vi "rsidr_core_global.vi"() -> ()   [LabVIEW 2020, in "Rohde&Schwarz RTx Oscilloscopes.lvlib"] (continued)
reference waveforms of all active channels, and activates the references. This action works only with single acquisition.\nThe channels are assigned to the references: C1 to R1, C2 to R2 and so on. If a channel is off, the assigned reference is also not active.\n\nAvailable Repeated Capabilities:\nNone\n\nRemote-control command(s):\nTRIGger:EVENt:REFSave"}, {"Level"=3, "Class Only"=FALSE, "Identifier"="RSRTX_ATTR_ACTIONS_ON_TRIGGER_PULSE_OUT", "Descriptive Name"="Actions On Trigger Pulse Out", "Data Type"=3, "Command"="TRIG:EVEN:TRIG", "Access"=2, "Range Table"="", "Read Callback"="", "Write Callback"="", "Supported Models"="", "Instrument Options"="", "Flags"=0, "Help"="If ON, the instrument generates a pulse on the Aux Out connector on trigger event. The acquisition is not delayed, the pulse generation runs asynchronously.\nTo set the pulse width and polarity of the trigger out pulse, use:\nRSRTX_ATTR_TRIGGER_OUT_PULSE_WIDTH\nRSRTX_ATTR_TRIGGER_OUT_POLARITY\n\nAvailable Repeated Capabilities:\nNone\n\nRemote-control command(s):\nTRIGger:EVENt:TRIGgerout"}, {"Level"=2, "Class Only"=TRUE, "Identifier"="", "Descriptive Name"="Trigger Out", "Data Type"=0, "Command"="", "Access"=0, "Range Table"="", "Read Callback"="", "Write Callback"="", "Supported Models"="", "Instrument Options"="", "Flags"=0, "Help"="Atributes configures the Trigger Out."}, {"Level"=3, "Class Only"=FALSE, "Identifier"="RSRTX_ATTR_TRIGGER_OUT_MODE", "Descriptive Name"="Trigger Out Mode", "Data Type"=0, "Command"="TRIG:OUT:MODE", "Access"=2, "Range Table"="rsrtx_rngTriggerOutMode", "Read Callback"="", "Write Callback"="", "Supported Models"="", "Instrument Options"="", "Flags"=0, "Help"="Defines wether and when a trigger out pulse is generated: never, on trigger event, or on mask violation.\n\nAvailable Repeated Capabilities:\nNone\n\nRemote-control command(s):\nTRIGger:OUT:MODE"}, {"Level"=3, "Class Only"=FALSE, "Identifier"="RSRTX_ATTR_TRIGGER_OUT_POLARITY", "Descriptive Name"="Trigger Out Polarity", "Data Type"=0, "Command"="TRIG:OUT:POL", "Access"=2, "Range Table"="rsrtx_rngPolarity", "Read Callback"="", "Write Callback"="", "Supported Models"="", "Instrument Options"="", "Flags"=0, "Help"="Sets the polarity of the trigger out pulse.\n\nAvailable Repeated Capabilities:\nNone\n\nRemote-control command(s):\nTRIGger:OUT:POLarity"}, {"Level"=3, "Class Only"=FALSE, "Identifier"="RSRTX_ATTR_TRIGGER_OUT_PULSE_WIDTH", "Descriptive Name"="Trigger Out Pulse Width", "Data Type"=1, "Command"="TRIG:OUT:PLEN", "Access"=2, "Range Table"="", "Read Callback"="", "Write Callback"="", "Supported Models"="", "Instrument Options"="", "Flags"=0, "Help"="Defines the pulse width of the trigger out pulse.\n\nAvailable Repeated Capabilities:\nNone\n\nRemote-control command(s):\nTRIGger:OUT:PLENgth"}, {"Level"=2, "Class Only"=TRUE, "Identifier"="", "Descriptive Name"="Runt", "Data Type"=0, "Command"="", "Access"=0, "Range Table"="", "Read Callback"="", "Write Callback"="", "Supported Models"="", "Instrument Options"="", "Flags"=0, "Help"="A runt is a pulse lower than normal in amplitude. The amplitude crosses the first\nthreshold twice in succession without crossing the second one. For example, this trig-\nger can detect logic, digital, and analog signals remaining below a specified threshold\namplitude because I/O ports are in undefined state."}, {"Level"=3, "Class Only"=FALSE, "Identifier"="RSRTX_ATTR_RUNT_TRIGGER_POLARITY", "Descriptive Name"="Runt Trigger Polarity", "Data Type"=0, "Command"="TRIG:A:RUNT:POL", "Access"=2, "Range Table"="rsrtx_rngPolarity", "Read Callback"="", "Write Callback"="", "Supported Models"="RTM|RTA", "Instrument Options"="", "Flags"=0, "Help"="Sets the polarity of a pulse, that is the direction of the first pulse slope.\n\nAvailable Repeated Capabilities:\nNone\n\nRemote-control command(s):\nTRIGger:A:RUNT:POLarity"}, {"Level"=3, "Class Only"=FALSE, "Identifier"="RSRTX_ATTR_RUNT_TRIGGER_WIDTH", "Descriptive Name"="Runt Trigger Width", "Data Type"=1, "Command"="TRIG:A:RUNT:WIDT", "Access"=2, "Range Table"="", "Read Callback"="", "Write Callback"="", "Supported Models"="RTM|RTA", "Instrument Options"="", "Flags"=0, "Help"="For the ranges WITHin and OUTSide, the <Time1> defines the center of a range which is defined by the limits +-<Delta>. For the ranges SHORter and LONGer, the width defines the maximum and minimum pulse width, respectively.\n\nAvailable Repeated Capabilities:\nNone\n\nRemote-control command(s):\nTRIGger:A:RUNT:WIDTh"}, {"Level"=3, "Class Only"=FALSE, "Identifier"="RSRTX_ATTR_RUNT_TRIGGER_DELTA", "Descriptive Name"="Runt Trigger Delta", "Data Type"=1, "Command"="TRIG:A:RUNT:DELT", "Access"=2, "Range Table"="", "Read Callback"="", "Write Callback"="", "Supported Models"="RTM|RTA", "Instrument Options"="", "Flags"=0, "Help"="Defines a range around the width value.\n\nAvailable Repeated Capabilities:\nNone\n\nRemote-control command(s):\nTRIGger:A:RUNT:DELTa"}, {"Level"=3, "Class Only"=FALSE, "Identifier"="RSRTX_ATTR_RUNT_TRIGGER_RANGE", "Descriptive Name"="Runt Trigger Range", "Data Type"=0, "Command"="TRIG:A:RUNT:RANG", "Access"=2, "Range Table"="rsrtx_rngWidthCondition", "Read Callback"="", "Write Callback"="", "Supported Models"="RTM|RTA", "Instrument Options"="", "Flags"=0, "Help"="Defines how the measured pulse width is compared with the given limit(s).\n\nAvailable Repeated Capabilities:\nNone\n\nRemote-control command(s):\nTRIGger:A:RUNT:RANGe"}, {"Level"=3, "Class Only"=TRUE, "Identifier"="", "Descriptive Name"="Channel", "Data Type"=0, "Command"="", "Access"=0, "Range Table"="", "Read Callback"="", "Write Callback"="", "Supported Models"="", "Instrument Options"="", "Flags"=0, "Help"="Attributes with channel repcap."}, {"Level"=4, "Class Only"=FALSE, "Identifier"="RSRTX_ATTR_RUNT_TRIGGER_LOWER_LEVEL", "Descriptive Name"="Runt Trigger Lower Level", "Data Type"=1, "Command"="TRIG:A:LEV{Channel}:RUNT:LOW", "Access"=2, "Range Table"="", "Read Callback"="", "Write Callback"="", "Supported Models"="RTM|RTA", "Instrument Options"="", "Flags"=0, "Help"="Set the lower voltage threshold. The instrument triggers if the amplitude crosses the first threshold twice in succession without crossing the second one.\n\nAvailable Repeated Capabilities:\nChannel: CH0, CH1, CH2, CH3, CH4, CHExt\r\n\nRemote-control command(s):\nTRIGger:A:LEVel<n>:RUNT:LOWer"}, {"Level"=4, "Class Only"=FALSE, "Identifier"="RSRTX_ATTR_RUNT_TRIGGER_UPPER_LEVEL", "Descriptive Name"="Runt Trigger Upper Level", "Data Type"=1, "Command"="TRIG:A:LEV{Channel}:RUNT:UPP", "Access"=2, "Range Table"="", "Read Callback"="", "Write Callback"="", "Supported Models"="RTM|RTA", "Instrument Options"="", "Flags"=0, "Help"="Set the upper voltage threshold. The instrument triggers if the amplitude crosses the first threshold twice in succession without crossing the second one.\n\nAvailable Repeated Capabilities:\nChannel: CH0, CH1, CH2, CH3, CH4, CHExt\r\n\nRemote-control command(s):\nTRIGger:A:LEVel<n>:RUNT:UPPer"}, {"Level"=2, "Class Only"=TRUE, "Identifier"="", "Descriptive Name"="Timeout", "Data Type"=0, "Command"="", "Access"=0, "Range Table"="", "Read Callback"="", "Write Callback"="", "Supported Models"="", "Instrument Options"="", "Flags"=0, "Help"="Configures the timeout trigger."}, {"Level"=3, "Class Only"=FALSE, "Identifier"="RSRTX_ATTR_TIMEOUT_TRIGGER_TIME", "Descriptive Name"="Timeout Trigger Time", "Data Type"=1, "Command"="TRIG:A:TIM:TIME", "Access"=2, "Range Table"="RsRtx_rngTimeoutTriggerTime", "Read Callback"="", "Write Callback"="", "Supported Models"="", "Instrument Options"="", "Flags"=0, "Help"="Sets the time limit for the timeout at which the instrument triggers.\n\nAvailable Repeated Capabilities:\nNone\n\nRemote-control command(s):\nTRIGger:A:TIMeout:TIME"}, {"Level"=3, "Class Only"=FALSE, "Identifier"="RSRTX_ATTR_TIMEOUT_TRIGGER_RANGE", "Descriptive Name"="Timeout Trigger Range", "Data Type"=0, "Command"="TRIG:A:TIM:RANG", "Access"=2, "Range Table"="RsRtx_rngTimeoutRange", "Read Callback"="", "Write Callback"="", "Supported Models"="", "Instrument Options"="", "Flags"=0, "Help"="Sets the relation of the signal level to the threshold.\n\nAvailable Repeated Capabilities:\nNone\n\nRemote-control command(s):\nTRIGger:A:TIMeout:RANGe"}, {"Level"=2, "Class Only"=TRUE, "Identifier"="", "Descriptive Name"="I2C", "Data Type"=0, "Command"="", "Access"=0, "Range Table"="", "Read Callback"="", "Write Callback"="", "Supported Models"="", "Instrument Options"="", "Flags"=0, "Help"="Atributes configures the Trigger for I2C protocol."}, {"Level"=3, "Class Only"=FALSE, "Identifier"="RSRTX_ATTR_PROTOCOL_I2C_TRIGGER_ACCESS", "Descriptive Name"="Protocol I2C Trigger Access", "Data Type"=0, "Command"="TRIG:A:I2C:ACC", "Access"=2, "Range Table"="rsrtx_rngProtocolI2CAccessBit", "Read Callback"="", "Write Callback"="", "Supported Models"="", "Instrument Options"="", "Flags"=0, "Help"="Toggles the trigger condition between Read and Write access of the master.\n\nAvailable Repeated Capabilities:\nNone\n\nRemote-control command(s):\nTRIGger:A:I2C:ACCess"}, {"Level"=3, "Class Only"=FALSE, "Identifier"="RSRTX_ATTR_PROTOCOL_I2C_TRIGGER_ADDRESS_TYPE", "Descriptive Name"="Protocol I2C Trigger Address Type", "Data Type"=0, "Command"="TRIG:A:I2C:AMOD", "Access"=2, "Range Table"="rsrtx_rngAddressLength", "Read Callback"="", "Write Callback"="", "Supported Models"="", "Instrument Options"="", "Flags"=0, "Help"="Sets the lenght of the slave address.\n\nAvailable Repeated Capabilities:\nNone\n\nRemote-control command(s):\nTRIGger:A:I2C:AMODe"}, {"Level"=3, "Class Only"=FALSE, "Identifier"="RSRTX_ATTR_PROTOCOL_I2C_TRIGGER_ADDRESS", "Descriptive Name"="Protocol I2C Trigger Address", "Data Type"=2, "Command"="TRIG:A:I2C:ADDR", "Access"=2, "Range Table"="", "Read Callback"="", "Write Callback"="", "Supported Models"="", "Instrument Options"="", "Flags"=0, "Help"="Sets the address of the slave device. The address can have 7 bits or 10 bits.\n\nAvailable Repeated Capabilities:\nNone\n\nRemote-control command(s):\nTRIGger:A:I2C:ADDRess"}, {"Level"=3, "Class Only"=FALSE, "Identifier"="RSRTX_ATTR_PROTOCOL_I2C_TRIGGER_MODE", "Descriptive Name"="Protocol I2C Trigger Mode", "Data Type"=0, "Command"="TRIG:A:I2C:MODE", "Access"=2, "Range Table"="rsrtx_rngProtocolI2CTriggerType", "Read Callback"="", "Write Callback"="", "Supported Models"="", "Instrument Options"="", "Flags"=0, "Help"="Specifies the trigger mode for I2C.\n\nAvailable Repeated Capabilities:\nNone\n\nRemote-control command(s):\nTRIGger:A:I2C:MODE"}, {"Level"=3, "Class Only"=FALSE, "Identifier"="RSRTX_ATTR_PROTOCOL_I2C_TRIGGER_CONDITION_LENGTH", "Descriptive Name"="Protocol I2C Trigger Condition Length", "Data Type"=0, "Command"="TRIG:A:I2C:PLEN", "Access"=2, "Range Table"="rsrtx_rngProtocolI2CPatternLength", "Read Callback"="", "Write Callback"="", "Supported Models"="", "Instrument Options"="", "Flags"=0, "Help"="Defines how many bytes are considered in the trigger condition. To set the pattern for these bytes, use RSRTX_ATTR_PROTOCOL_I2C_TRIGGER_BIT_PATTERN.\n\nAvailable Repeated Capabilities:\nNone\n\nRemote-control command(s):\nTRIGger:A:I2C:PLENgth"}, {"Level"=3, "Class Only"=FALSE, "Identifier"="RSRTX_ATTR_PROTOCOL_I2C_TRIGGER_BIT_PATTERN", "Descriptive Name"="Protocol I2C Trigger Bit Pattern", "Data Type"=2, "Command"="TRIG:A:I2C:PATT", "Access"=2, "Range Table"="", "Read Callback"="", "Write Callback"="", "Supported Models"="", "Instrument Options"="", "Flags"=0, "Help"="Defines the bit pattern as trigger condition. Make sure that the correct pattern length has been defined before with RSRTX_ATTR_PROTOCOL_I2C_TRIGGER_CONDITION_LENGTH. SBinary pattern with max. 24 bit. Characters 0, 1, and X are allowed.\n\nAvailable Repeated Capabilities:\nNone\n\nRemote-control command(s):\nTRIGger:A:I2C:PATTern"}, {"Level"=3, "Class Only"=FALSE, "Identifier"="RSRTX_ATTR_PROTOCOL_I2C_TRIGGER_FIRST_BYTE_OFFSET", "Descriptive Name"="Protocol I2C Trigger First Byte Offset", "Data Type"=0, "Command"="TRIG:A:I2C:POFF", "Access"=2, "Range Table"="rsrtx_rngFirstBitOffset", "Read Callback"="", "Write Callback"="", "Supported Models"="", "Instrument Options"="", "Flags"=0, "Help"="Sets the number of bytes before the first byte of interest, relating to the end of the address bytes.\n\nAvailable Repeated Capabilities:\nNone\n\nRemote-control command(s):\nTRIGger:A:I2C:POFFset"}, {"Level"=2, "Class Only"=TRUE, "Identifier"="", "Descriptive Name"="SPI", "Data Type"=0, "Command"="", "Access"=0, "Range Table"="", "Read Callback"="", "Write Callback"="", "Supported Models"="", "Instrument Options"="", "Flags"=0, "Help"="Atributes configures the Trigger for SPI protocol."}, {"Level"=3, "Class Only"=FALSE, "Identifier"="RSRTX_ATTR_PROTOCOL_SPI_TRIGGER_MODE", "Descriptive Name"="Protocol SPI Trigger Mode", "Data Type"=0, "Command"="TRIG:A:SPI:MODE", "Access"=2, "Range Table"="rsrtx_rngProtocolSPITriggerType", "Read Callback"="", "Write Callback"="", "Supported Models"="", "Instrument Options"="", "Flags"=0, "Help"="Specifies the trigger mode for SPI/SSPI protocols.\n\nAvailable Repeated Capabilities:\nNone\n\nRemote-control command(s):\nTRIGger:A:SPI:MODE"}, {"Level"=3, "Class Only"=FALSE, "Identifier"="RSRTX_ATTR_PROTOCOL_SPI_TRIGGER_SOURCE", "Descriptive Name"="Protocol SPI Trigger Source", "Data Type"=0, "Command"="TRIG:A:SOUR:SPI", "Access"=2, "Range Table"="rsrtx_rngProtocolSPITriggerSource", "Read Callback"="", "Write Callback"="", "Supported Models"="RTM|RTA", "Instrument Options"="", "Flags"=0, "Help"="Selects the trigger source.\n\nAvailable Repeated Capabilities:\nNone\n\nRemote-control command(s):\nTRIGger:A:SOURce:SPI"}, {"Level"=3, "Class Only"=FALSE, "Identifier"="RSRTX_ATTR_PROTOCOL_SPI_TRIGGER_OFFSET", "Descriptive Name"="Protocol SPI Trigger Offset", "Data Type"=0, "Command"="TRIG:A:SPI:POFF", "Access"=2, "Range Table"="rsrtx_rngFirstBitOffset", "Read Callback"="", "Write Callback"="", "Supported Models"="", "Instrument Options"="", "Flags"=0, "Help"="Sets the number of bits before the first bit of the pattern.\n\nAvailable Repeated Capabilities:\nNone\n\nRemote-control command(s):\nTRIGger:A:SPI:POFFset"}, {"Level"=3, "Class Only"=FALSE, "Identifier"="RSRTX_ATTR_PROTOCOL_SPI_BIT_PATTERN_LENGTH", "Descriptive Name"="Protocol SPI Bit Pattern Length", "Data Type"=0, "Command"="TRIG:A:SPI:PLEN", "Access"=2, "Range Table"="rsrtx_rngSPIWordLength", "Read Callback"="", "Write Callback"="", "Supported Models"="", "Instrument Options"="", "Flags"=0, "Help"="Defines how many bits build up the serial pattern.\n\nAvailable Repeated Capabilities:\nNone\n\nRemote-control command(s):\nTRIGger:A:SPI:PLENgth"}, {"Level"=3, "Class Only"=FALSE, "Identifier"="RSRTX_ATTR_PROTOCOL_SPI_BIT_PATTERN", "Descriptive Name"="Protocol SPI Bit Pattern", "Data Type"=2, "Command"="TRIG:A:SPI:PATT", "Access"=2, "Range Table"="", "Read Callback"="", "Write Callback"="", "Supported Models"="", "Instrument Options"="", "Flags"=0, "Help"="Defines the bit pattern as trigger condition. The pattern length is adjusted to the number of bits defined in the pattern.\n\nAvailable Repeated Capabilities:\nNone\n\nRemote-control command(s):\nTRIGger:A:SPI:PATTern"}, {"Level"=2, "Class Only"=TRUE, "Identifier"="", "Descriptive Name"="UART", "Data Type"=0, "Command"="", "Access"=0, "Range Table"="", "Read Callback"="", "Write Callback"="", "Supported Models"="", "Instrument Options"="", "Flags"=0, "Help"="Atributes configures the Trigger for UART protocol."}, {"Level"=3, "Class Only"=FALSE, "Identifier"="RSRTX_ATTR_PROTOCOL_UART_TRIGGER_MODE", "Descriptive Name"="Protocol UART Trigger Mode", "Data Type"=0, "Command"="TRIG:A:UART:MODE", "Access"=2, "Range Table"="rsrtx_rngProtocolUARTTriggerType", "Read Callback"="", "Write Callback"="", "Supported Models"="", "Instrument Options"="", "Flags"=0, "Help"="Specifies the trigger mode for UART/RS-232 interfaces.\n\nAvailable Repeated Capabilities:\nNone\n\nRemote-control command(s):\nTRIGger:A:UART:MODE"}, {"Level"=3, "Class Only"=FALSE, "Identifier"="RSRTX_ATTR_PROTOCOL_UART_TRIGGER_SOURCE", "Descriptive Name"="Protocol UART Trigger Source", "Data Type"=0, "Command"="TRIG:A:SOUR:UART", "Access"=2, "Range Table"="RsRtx_rngUARTTriggerSource", "Read Callback"="", "Write Callback"="", "Supported Models"="RTM|RTA", "Instrument Options"="", "Flags"=0, "Help"="Configures the UART trigger source\n\nAvailable Repeated Capabilities:\nNone\n\nRemote-control command(s):\nTRIGger:A:SOURce:UART"}, {"Level"=3, "Class Only"=FALSE, "Identifier"="RSRTX_ATTR_PROTOCOL_UART_TRIGGER_DATA_PATTERN", "Descriptive Name"="Protocol UART Trigger Data Pattern", "Data Type"=2, "Command"="TRIG:A:UART:PATT", "Access"=2, "Range Table"="", "Read Callback"="", "Write Callback"="", "Supported Models"="", "Instrument Options"="", "Flags"=0, "Help"="Defines the bit pattern as trigger condition.\n\nAvailable Repeated Capabilities:\nNone\n\nRemote-control command(s):\nTRIGger:A:UART:PATTern"}, {"Level"=3, "Class Only"=FALSE, "Identifier"="RSRTX_ATTR_PROTOCOL_UART_TRIGGER_DATA_POSITION_INDEX_MIN", "Descriptive Name"="Protocol UART Trigger Data Position Index Min", "Data Type"=0, "Command"="TRIG:A:UART:POFF", "Access"=2, "Range Table"="rsrtx_rngFirstBitOffset", "Read Callback"="", "Write Callback"="", "Supported Models"="", "Instrument Options"="", "Flags"=0, "Help"="Sets the number of symbols before the first symbol of the pattern.\n\nAvailable Repeated Capabilities:\nNone\n\nRemote-control command(s):\nTRIGger:A:UART:POFFset"}, {"Level"=3, "Class Only"=FALSE, "Identifier"="RSRTX_ATTR_PROTOCOL_UART_TRIGGER_CONDITION_LENGTH", "Descriptive Name"="Protocol UART Trigger Condition Length", "Data Type"=0, "Command"="TRIG:A:UART:PLEN", "Access"=2, "Range Table"="rsrtx_rngUartLength", "Read Callback"="", "Write Callback"="", "Supported Models"="", "Instrument Options"="", "Flags"=0, "Help"="Defines how many symbols build up the serial pattern.\n\nAvailable Repeated Capabilities:\nNone\n\nRemote-control command(s):\nTRIGger:A:UART:PLENgth"}, {"Level"=2, "Class Only"=TRUE, "Identifier"="", "Descriptive Name"="LIN", "Data Type"=0, "Command"="", "Access"=0, "Range Table"="", "Read Callback"="", "Write Callback"="", "Supported Models"="", "Instrument Options"="", "Flags"=0, "Help"="Atributes configures the Trigger for LIN protocol."}, {"Level"=3, "Class Only"=FALSE, "Identifier"="RSRTX_ATTR_PROTOCOL_LIN_TRIGGER_MODE", "Descriptive Name"="Protocol LIN Trigger Mode", "Data Type"=0, "Command"="TRIG:A:LIN:TYPE", "Access"=2, "Range Table"="rsrtx_rngProtocolLINTriggerMode", "Read Callback"="", "Write Callback"="", "Supported Models"="", "Instrument Options"="K3", "Flags"=0, "Help"="Selects the trigger type for LIN analysis.\n\nAvailable Repeated Capabilities:\nNone\n\nRemote-control command(s):\nTRIGger:A:LIN:TYPE"}, {"Level"=3, "Class Only"=FALSE, "Identifier"="RSRTX_ATTR_PROTOCOL_LIN_TRIGGER_CONDITION_ID", "Descriptive Name"="Protocol LIN Trigger Condition ID", "Data Type"=0, "Command"="TRIG:A:LIN:ICON", "Access"=2, "Range Table"="rsrtx_rngProtocolCondition", "Read Callback"="", "Write Callback"="", "Supported Models"="", "Instrument Options"="K3", "Flags"=0, "Help"="Sets the condition.\n\nAvailable Repeated Capabilities:\nNone\n\nRemote-control command(s):\nTRIGger:A:LIN:ICONdition"}, {"Level"=3, "Class Only"=FALSE, "Identifier"="RSRTX_ATTR_PROTOCOL_LIN_TRIGGER_CONDITION_DATA", "Descriptive Name"="Protocol LIN Trigger Condition Data", "Data Type"=0, "Command"="TRIG:A:LIN:DCON", "Access"=2, "Range Table"="rsrtx_rngProtocolCondition", "Read Callback"="", "Write Callback"="", "Supported Models"="", "Instrument Options"="K3", "Flags"=0, "Help"="Sets the condition.\n\nAvailable Repeated Capabilities:\nNone\n\nRemote-control command(s):\nTRIGger:A:LIN:DCONdition"}, {"Level"=3, "Class Only"=FALSE, "Identifier"="RSRTX_ATTR_PROTOCOL_LIN_TRIGGER_ID_PATTERN", "Descriptive Name"="Protocol LIN Trigger ID Pattern", "Data Type"=2, "Command"="TRIG:A:LIN:IDEN", "Access"=2, "Range Table"="", "Read Callback"="", "Write Callback"="", "Supported Models"="", "Instrument Options"="K3", "Flags"=0, "Help"="Defines the identifier pattern. Relevant if RSRTX_ATTR_PROTOCOL_LIN_TRIGGER_MODE is set to ID or IDDT.\n\nAvailable Repeated Capabilities:\nNone\n\nRemote-control command(s):\nTRIGger:A:LIN:IDENtifier"}, {"Level"=3, "Class Only"=FALSE, "Identifier"="RSRTX_ATTR_PROTOCOL_LIN_TRIGGER_DATA_LENGTH", "Descriptive Name"="Protocol LIN Trigger Data Length", "Data Type"=0, "Command"="TRIG:A:LIN:DLEN", "Access"=2, "Range Table"="rsrtx_rngProtocolLINDataLength", "Read Callback"="", "Write Callback"="", "Supported Models"="", "Instrument Options"="K3", "Flags"=0, "Help"="Defines the length of the data pattern - the number of bytes in the pattern.\n\nAvailable Repeated Capabilities:\nNone\n\nRemote-control command(s):\nTRIGger:A:LIN:DLENgth"}, {"Level"=3, "Class Only"=FALSE, "Identifier"="RSRTX_ATTR_PROTOCOL_LIN_TRIGGER_DATA_PATTERN", "Descriptive Name"="Protocol LIN Trigger Data Pattern", "Data Type"=2, "Command"="TRIG:A:LIN:DATA", "Access"=2, "Range Table"="", "Read Callback"="", "Write Callback"="", "Supported Models"="", "Instrument Options"="K3", "Flags"=0, "Help"="Defines the data pattern. The number of bytes in  the data pattern is defined with RSRTX_ATTR_PROTOCOL_LIN_TRIGGER_DATA_LENGTH.\n\nRelevant if RSRTX_ATTR_PROTOCOL_LIN_TRIGGER_MODE is set to IDDT.\n\nAvailable Repeated Capabilities:\nNone\n\nRemote-control command(s):\nTRIGger:A:LIN:DATA"}, {"Level"=3, "Class Only"=FALSE, "Identifier"="RSRTX_ATTR_PROTOCOL_LIN_TRIGGER_ERROR_CHECKSUM", "Descriptive Name"="Protocol LIN Trigger Error Checksum", "Data Type"=3, "Command"="TRIG:A:LIN:CHKS", "Access"=2, "Range Table"="", "Read Callback"="", "Write Callback"="", "Supported Models"="", "Instrument Options"="K3", "Flags"=0, "Help"="Configures conditions for Error Condition trigger.\n\nAvailable Repeated Capabilities:\nNone\n\nRemote-control command(s):\nTRIGger:A:LIN:CHKSerror"}, {"Level"=3, "Class Only"=FALSE, "Identifier"="RSRTX_ATTR_PROTOCOL_LIN_TRIGGER_ERROR_PARITY", "Descriptive Name"="Protocol LIN Trigger Error Parity", "Data Type"=3, "Command"="TRIG:A:LIN:IPER", "Access"=2, "Range Table"="", "Read Callback"="", "Write Callback"="", "Supported Models"="", "Instrument Options"="K3", "Flags"=0, "Help"="Configures conditions for Error Condition trigger.\n\nAvailable Repeated Capabilities:\nNone\n\nRemote-control command(s):\nTRIGger:A:LIN:IPERror"}, {"Level"=3, "Class Only"=FALSE, "Identifier"="RSRTX_ATTR_PROTOCOL_LIN_TRIGGER_ERROR_SYNC", "Descriptive Name"="Protocol LIN Trigger Error Sync", "Data Type"=3, "Command"="TRIG:A:LIN:SYER", "Access"=2, "Range Table"="", "Read Callback"="", "Write Callback"="", "Supported Models"="", "Instrument Options"="K3", "Flags"=0, "Help"="Configures conditions for Error Condition trigger.\n\nAvailable Repeated Capabilities:\nNone\n\nRemote-control command(s):\nTRIGger:A:LIN:SYERror"}, {"Level"=2, "Class Only"=TRUE, "Identifier"="", "Descriptive Name"="CAN", "Data Type"=0, "Command"="", "Access"=0, "Range Table"="", "Read Callback"="", "Write Callback"="", "Supported Models"="", "Instrument Options"="", "Flags"=0, "Help"="Atributes configures the Trigger for CAN protocol."}, {"Level"=3, "Class Only"=FALSE, "Identifier"="RSRTX_ATTR_PROTOCOL_CAN_TRIGGER_MODE", "Descriptive Name"="Protocol CAN Trigger Mode", "Data Type"=0, "Command"="TRIG:A:CAN:TYPE", "Access"=2, "Range Table"="rsrtx_rngProtocolCANTriggerMode", "Read Callback"="", "Write Callback"="", "Supported Models"="", "Instrument Options"="K3", "Flags"=0, "Help"="Selects the trigger type for LIN analysis.\n\nAvailable Repeated Capabilities:\nNone\n\nRemote-control command(s):\nTRIGger:A:CAN:TYPE"}, {"Level"=3, "Class Only"=FALSE, "Identifier"="RSRTX_ATTR_PROTOCOL_CAN_TRIGGER_FRAME_TYPE", "Descriptive Name"="Protocol CAN Trigger Frame Type", "Data Type"=0, "Command"="TRIG:A:CAN:FTYP", "Access"=2, "Range Table"="rsrtx_rngProtocolCANTriggerFrameType", "Read Callback"="", "Write Callback"="", "Supported Models"="", "Instrument Options"="", "Flags"=0, "Help"="Selects the frame type which will be used as trigger condition.\n\nAvailable Repeated Capabilities:\nNone\n\nRemote-control command(s):\nTRIGger:A:CAN:FTYPe"}, {"Level"=3, "Class Only"=FALSE, "Identifier"="RSRTX_ATTR_PROTOCOL_CAN_TRIGGER_CONDITION_ID", "Descriptive Name"="Protocol CAN Trigger Condition ID", "Data Type"=0, "Command"="TRIG:A:CAN:ICON", "Access"=2, "Range Table"="rsrtx_rngProtocolCondition", "Read Callback"="", "Write Callback"="", "Supported Models"="", "Instrument Options"="K3", "Flags"=0, "Help"="Sets the condition.\n\nAvailable Repeated Capabilities:\nNone\n\nRemote-control command(s):\nTRIGger:A:CAN:ICONdition"}, {"Level"=3, "Class Only"=FALSE, "Identifier"="RSRTX_ATTR_PROTOCOL_CAN_TRIGGER_CONDITION_DATA", "Descriptive Name"="Protocol CAN Trigger Condition Data", "Data Type"=0, "Command"="TRIG:A:CAN:DCON", "Access"=2, "Range Table"="rsrtx_rngProtocolCondition", "Read Callback"="", "Write Callback"="", "Supported Models"="", "Instrument Options"="K3", "Flags"=0, "Help"="Sets the condition.\n\nAvailable Repeated Capabilities:\nNone\n\nRemote-control command(s):\nTRIGger:A:CAN:DCONdition"}, {"Level"=3, "Class Only"=FALSE, "Identifier"="RSRTX_ATTR_PROTOCOL_CAN_TRIGGER_ID_TYPE", "Descriptive Name"="Protocol CAN Trigger ID Type", "Data Type"=0, "Command"="TRIG:A:CAN:ITYP", "Access"=2, "Range Table"="rsrtx_rngProtocolCANIDType", "Read Callback"="", "Write Callback"="", "Supported Models"="", "Instrument Options"="K3", "Flags"=0, "Help"="Selects the format of data and remote frames.\n\nAvailable Repeated Capabilities:\nNone\n\nRemote-control command(s):\nTRIGger:A:CAN:ITYPe"}, {"Level"=3, "Class Only"=FALSE, "Identifier"="RSRTX_ATTR_PROTOCOL_CAN_TRIGGER_ID_PATTERN", "Descriptive Name"="Protocol CAN Trigger ID Pattern", "Data Type"=2, "Command"="TRIG:A:CAN:IDEN", "Access"=2, "Range Table"="", "Read Callback"="", "Write Callback"="", "Supported Models"="", "Instrument Options"="K3", "Flags"=0, "Help"="Defines the identifier pattern. The pattern length is defined with RSRTX_ATTR_PROTOCOL_CAN_TRIGGER_ID_TYPE.\n\nRelevant if RSRTX_ATTR_PROTOCOL_CAN_TRIGGER_MODE is set to ID or IDDT.\n\nAvailable Repeated Capabilities:\nNone\n\nRemote-control command(s):\nTRIGger:A:CAN:IDENtifier"}, {"Level"=3, "Class Only"=FALSE, "Identifier"="RSRTX_ATTR_PROTOCOL_CAN_TRIGGER_DATA_LENGTH", "Descriptive Name"="Protocol CAN Trigger Data Length", "Data Type"=0, "Command"="TRIG:A:CAN:DLC", "Access"=2, "Range Table"="rsrtx_rngProtocolCANDataLength", "Read Callback"="", "Write Callback"="", "Supported Models"="", "Instrument Options"="K3", "Flags"=0, "Help"="Defines the length of the data pattern - the number of bytes in the pattern.\n\nAvailable Repeated Capabilities:\nNone\n\nRemote-control command(s):\nTRIGger:A:CAN:DLC"}, {"Level"=3, "Class Only"=FALSE, "Identifier"="RSRTX_ATTR_PROTOCOL_CAN_TRIGGER_DATA_PATTERN", "Descriptive Name"="Protocol CAN Trigger Data Pattern", "Data Type"=2, "Command"="TRIG:A:CAN:DATA", "Access"=2, "Range Table"="", "Read Callback"="", "Write Callback"="", "Supported Models"="", "Instrument Options"="K3", "Flags"=0, "Help"="Defines the data pattern. The number of bytes in the data pattern is defined with RSRTX_ATTR_PROTOCOL_CAN_TRIGGER_DATA_LENGTH.\n\nRelevant if RSRTX_ATTR_PROTOCOL_CAN_TRIGGER_MODE is set to IDDT.\n\nAvailable Repeated Capabilities:\nNone\n\nRemote-control command(s):\nTRIGger:A:CAN:DATA"}, {"Level"=3, "Class Only"=FALSE, "Identifier"="RSRTX_ATTR_PROTOCOL_CAN_TRIGGER_ERROR_CRC", "Descriptive Name"="Protocol CAN Trigger Error CRC", "Data Type"=3, "Command"="TRIG:A:CAN:CRC", "Access"=2, "Range Table"="", "Read Callback"="", "Write Callback"="", "Supported Models"="", "Instrument Options"="K3", "Flags"=0, "Help"="Configures conditions for Error Condition trigger.\n\nAvailable Repeated Capabilities:\nNone\n\nRemote-control command(s):\nTRIGger:A:CAN:CRCerror"}, {"Level"=3, "Class Only"=FALSE, "Identifier"="RSRTX_ATTR_PROTOCOL_CAN_TRIGGER_ERROR_STUFFING", "Descriptive Name"="Protocol CAN Trigger Error Stuffing", "Data Type"=3, "Command"="TRIG:A:CAN:BITS", "Access"=2, "Range Table"="", "Read Callback"="", "Write Callback"="", "Supported Models"="", "Instrument Options"="K3", "Flags"=0, "Help"="Configures conditions for Error Condition trigger.\n\nAvailable Repeated Capabilities:\nNone\n\nRemote-control command(s):\nTRIGger:A:CAN:BITSterror"}, {"Level"=3, "Class Only"=FALSE, "Identifier"="RSRTX_ATTR_PROTOCOL_CAN_TRIGGER_ERROR_FORM", "Descriptive Name"="Protocol CAN Trigger Error Form", "Data Type"=3, "Command"="TRIG:A:CAN:FORM", "Access"=2, "Range Table"="", "Read Callback"="", "Write Callback"="", "Supported Models"="", "Instrument Options"="K3", "Flags"=0, "Help"="Configures conditions for Error Condition trigger.\n\nAvailable Repeated Capabilities:\nNone\n\nRemote-control command(s):\nTRIGger:A:CAN:FORMerror"}, {"Level"=3, "Class Only"=FALSE, "Identifier"="RSRTX_ATTR_PROTOCOL_CAN_TRIGGER_ERROR_ACK", "Descriptive Name"="Protocol CAN Trigger Error Ack", "Data Type"=3, "Command"="TRIG:A:CAN:ACK", "Access"=2, "Range Table"="", "Read Callback"="", "Write Callback"="", "Supported Models"="", "Instrument Options"="K3", "Flags"=0, "Help"="Configures conditions for Error Condition trigger.\n\nAvailable Repeated Capabilities:\nNone\n\nRemote-control command(s):\nTRIGger:A:CAN:ACKerror"}, {"Level"=2, "Class Only"=TRUE, "Identifier"="", "Descriptive Name"="Audio Signals", "Data Type"=0, "Command"="", "Access"=0, "Range Table"="", "Read Callback"="", "Write Callback"="", "Supported Models"="", "Instrument Options"="", "Flags"=0, "Help"="Configures Audio Signals trigger settings."}, {"Level"=3, "Class Only"=FALSE, "Identifier"="RSRTX_ATTR_PROTOCOL_AUDIO_TRIGGER_TYPE", "Descriptive Name"="Protocol Audio Trigger Type", "Data Type"=0, "Command"="TRIG:A:I2S:TYPE", "Access"=2, "Range Table"="rsrtx_rngAudioTriggerType", "Read Callback"="", "Write Callback"="", "Supported Models"="RTM|RTA", "Instrument Options"="", "Flags"=0, "Help"="Selects the trigger type.\n\nAvailable Repeated Capabilities:\nNone\n\nRemote-control command(s):\nTRIGger:A:I2S:TYPE"}, {"Level"=3, "Class Only"=FALSE, "Identifier"="RSRTX_ATTR_PROTOCOL_AUDIO_TRIGGER_WINDOW_LENGTH", "Descriptive Name"="Protocol Audio Trigger Window Length", "Data Type"=0, "Command"="TRIG:A:I2S:WIND:LENG", "Access"=2, "Range Table"="rsrtx_rngProtocolAudioWindowLength", "Read Callback"="", "Write Callback"="", "Supported Models"="RTM|RTA", "Instrument Options"="", "Flags"=0, "Help"="Sets the number of words that is used as time limit for the Window trigger type.\n\nAvailable Repeated Capabilities:\nNone\n\nRemote-control command(s):\nTRIGger:A:I2S:WINDow:LENGth"}, {"Level"=3, "Class Only"=FALSE, "Identifier"="RSRTX_ATTR_PROTOCOL_AUDIO_TRIGGER_WORD_SELECT_SLOPE", "Descriptive Name"="Protocol Audio Trigger Word Select Slope", "Data Type"=0, "Command"="TRIG:A:I2S:WSEL:SLOP", "Access"=2, "Range Table"="rsrtx_rngPolarity", "Read Callback"="", "Write Callback"="", "Supported Models"="RTM|RTA", "Instrument Options"="", "Flags"=0, "Help"="Sets the edge of the WS or FSYNC signal as trigger condition.\n\nAvailable Repeated Capabilities:\nNone\n\nRemote-control command(s):\nTRIGger:A:I2S:WSELect:SLOPe"}, {"Level"=3, "Class Only"=FALSE, "Identifier"="RSRTX_ATTR_PROTOCOL_AUDIO_TRIGGER_RIGHT_CONDITION", "Descriptive Name"="Protocol Audio Trigger Right Condition", "Data Type"=0, "Command"="TRIG:A:I2S:CHAN:RIGH:COND", "Access"=2, "Range Table"="rsrtx_rngAudioTriggerCondition", "Read Callback"="", "Write Callback"="", "Supported Models"="RTM|RTA", "Instrument Options"="", "Flags"=0, "Help"="Define the operators for comparison of the decoded data words with the specified data words on the specified channel.\n\nAvailable Repeated Capabilities:\nNone\n\nRemote-control command(s):\nTRIGger:A:I2S:CHANnel:RIGHt:CONDition"}, {"Level"=3, "Class Only"=FALSE, "Identifier"="RSRTX_ATTR_PROTOCOL_AUDIO_TRIGGER_RIGHT_MINIMUM", "Descriptive Name"="Protocol Audio Trigger Right Minimum", "Data Type"=0, "Command"="TRIG:A:I2S:CHAN:RIGH:DMIN", "Access"=2, "Range Table"="", "Read Callback"="", "Write Callback"="", "Supported Models"="RTM|RTA", "Instrument Options"="", "Flags"=0, "Help"="Specifies the data word to be found, or the minimum value of a data range.\n\nAvailable Repeated Capabilities:\nNone\n\nRemote-control command(s):\nTRIGger:A:I2S:CHANnel:RIGHt:DMIN"}, {"Level"=3, "Class Only"=FALSE, "Identifier"="RSRTX_ATTR_PROTOCOL_AUDIO_TRIGGER_RIGHT_MAXIMUM", "Descriptive Name"="Protocol Audio Trigger Right Maximum", "Data Type"=0, "Command"="TRIG:A:I2S:CHAN:RIGH:DMAX", "Access"=2, "Range Table"="", "Read Callback"="", "Write Callback"="", "Supported Models"="RTM|RTA", "Instrument Options"="", "Flags"=0, "Help"="Specifies the maximum data value to be found.\n\nAvailable Repeated Capabilities:\nNone\n\nRemote-control command(s):\nTRIGger:A:I2S:CHANnel:RIGHt:DMAX"}, {"Level"=3, "Class Only"=FALSE, "Identifier"="RSRTX_ATTR_PROTOCOL_AUDIO_TRIGGER_LEFT_CONDITION", "Descriptive Name"="Protocol Audio Trigger Left Condition", "Data Type"=0, "Command"="TRIG:A:I2S:CHAN:LEFT:COND", "Access"=2, "Range Table"="rsrtx_rngAudioTriggerCondition", "Read Callback"="", "Write Callback"="", "Supported Models"="RTM|RTA", "Instrument Options"="", "Flags"=0, "Help"="Define the operators for comparison of the decoded data words with the specified data words on the specified channel.\n\nAvailable Repeated Capabilities:\nNone\n\nRemote-control command(s):\nTRIGger:A:I2S:CHANnel:LEFT:CONDition"}, {"Level"=3, "Class Only"=FALSE, "Identifier"="RSRTX_ATTR_PROTOCOL_AUDIO_TRIGGER_LEFT_MINIMUM", "Descriptive Name"="Protocol Audio Trigger Left Minimum", "Data Type"=0, "Command"="TRIG:A:I2S:CHAN:LEFT:DMIN", "Access"=2, "Range Table"="", "Read Callback"="", "Write Callback"="", "Supported Models"="RTM|RTA", "Instrument Options"="", "Flags"=0, "Help"="Specifies the data word to be found, or the minimum value of a data range.\n\nAvailable Repeated Capabilities:\nNone\n\nRemote-control command(s):\nTRIGger:A:I2S:CHANnel:LEFT:DMIN"}, {"Level"=3, "Class Only"=FALSE, "Identifier"="RSRTX_ATTR_PROTOCOL_AUDIO_TRIGGER_LEFT_MAXIMUM", "Descriptive Name"="Protocol Audio Trigger Left Maximum", "Data Type"=0, "Command"="TRIG:A:I2S:CHAN:LEFT:DMAX", "Access"=2, "Range Table"="", "Read Callback"="", "Write Callback"="", "Supported Models"="RTM|RTA", "Instrument Options"="", "Flags"=0, "Help"="Specifies the maximum data value to be found.\n\nAvailable Repeated Capabilities:\nNone\n\nRemote-control command(s):\nTRIGger:A:I2S:CHANnel:LEFT:DMAX"}, {"Level"=3, "Class Only"=FALSE, "Identifier"="RSRTX_ATTR_PROTOCOL_AUDIO_TRIGGER_COMBINATION", "Descriptive Name"="Protocol Audio Trigger Combination", "Data Type"=0, "Command"="TRIG:A:I2S:FUNC", "Access"=2, "Range Table"="rsrtx_rngAudioTriggerCombination", "Read Callback"="", "Write Callback"="", "Supported Models"="RTM|RTA", "Instrument Options"="", "Flags"=0, "Help"="Sets the logical combination to trigger on data words on different channels. The instrument triggers if all conditions are met inside one frame.\n\nAvailable Repeated Capabilities:\nNone\n\nRemote-control command(s):\nTRIGger:A:I2S:FUNCtion"}, {"Level"=3, "Class Only"=TRUE, "Identifier"="", "Descriptive Name"="Track Channel", "Data Type"=0, "Command"="", "Access"=0, "Range Table"="", "Read Callback"="", "Write Callback"="", "Supported Models"="", "Instrument Options"="", "Flags"=0, "Help"="Selects the track channel."}, {"Level"=4, "Class Only"=FALSE, "Identifier"="RSRTX_ATTR_PROTOCOL_AUDIO_TRIGGER_CHANNEL_CONDITION", "Descriptive Name"="Protocol Audio Trigger Channel Condition", "Data Type"=0, "Command"="TRIG:A:I2S:CHAN:TDM{TDMChannel}:COND", "Access"=2, "Range Table"="rsrtx_rngAudioTriggerCondition", "Read Callback"="", "Write Callback"="", "Supported Models"="RTM|RTA", "Instrument Options"="", "Flags"=0, "Help"="Define the operators for comparison of the decoded data words with the specified data words on the specified channel.\n\nAvailable Repeated Capabilities:\nTDMChannel: TDM0, TDM1, TDM2, TDM3, TDM4, TDM5, TDM6, TDM7, TDM8\r\n\nRemote-control command(s):\nTRIGger:A:I2S:CHANnel:TDM<n>:CONDition"}, {"Level"=4, "Class Only"=FALSE, "Identifier"="RSRTX_ATTR_PROTOCOL_AUDIO_TRIGGER_CHANNEL_MINIMUM", "Descriptive Name"="Protocol Audio Trigger Channel Minimum", "Data Type"=0, "Command"="TRIG:A:I2S:CHAN:TDM{TDMChannel}:DMIN", "Access"=2, "Range Table"="", "Read Callback"="", "Write Callback"="", "Supported Models"="RTM|RTA", "Instrument Options"="", "Flags"=0, "Help"="Specifies the data word to be found, or the minimum value of a data range.\n\nAvailable Repeated Capabilities:\nTDMChannel: TDM0, TDM1, TDM2, TDM3, TDM4, TDM5, TDM6, TDM7, TDM8\r\n\nRemote-control command(s):\nTRIGger:A:I2S:CHANnel:TDM<n>:DMIN"}, {"Level"=4, "Class Only"=FALSE, "Identifier"="RSRTX_ATTR_PROTOCOL_AUDIO_TRIGGER_CHANNEL_MAXIMUM", "Descriptive Name"="Protocol Audio Trigger Channel Maximum", "Data Type"=0, "Command"="TRIG:A:I2S:CHAN:TDM{TDMChannel}:DMAX", "Access"=2, "Range Table"="", "Read Callback"="", "Write Callback"="", "Supported Models"="RTM|RTA", "Instrument Options"="", "Flags"=0, "Help"="Specifies the maximum data value to be found.\n\nAvailable Repeated Capabilities:\nTDMChannel: TDM0, TDM1, TDM2, TDM3, TDM4, TDM5, TDM6, TDM7, TDM8\r\n\nRemote-control command(s):\nTRIGger:A:I2S:CHANnel:TDM<n>:DMAX"}, {"Level"=2, "Class Only"=TRUE, "Identifier"="", "Descriptive Name"="MILSTD", "Data Type"=0, "Command"="", "Access"=0, "Range Table"="", "Read Callback"="", "Write Callback"="", "Supported Models"="", "Instrument Options"="", "Flags"=0, "Help"="The MIL-STD-1553 specification defines the characteristics of a serial data bus originally designed for use in the military avionics. Nowadays it is also used in spacecraft on-board data handling."}, {"Level"=3, "Class Only"=FALSE, "Identifier"="RSRTX_ATTR_MILSTD_TRIGGER_TYPE", "Descriptive Name"="MILSTD Trigger Type", "Data Type"=0, "Command"="TRIG:A:MILS:TYPE", "Access"=2, "Range Table"="rsrtx_rngMILSTDTriggerType", "Read Callback"="", "Write Callback"="", "Supported Models"="RTM|RTA", "Instrument Options"="", "Flags"=0, "Help"="Selects the trigger type.\n\nAvailable Repeated Capabilities:\nNone\n\nRemote-control command(s):\nTRIGger:A:MILStd:TYPE"}, {"Level"=3, "Class Only"=FALSE, "Identifier"="RSRTX_ATTR_MILSTD_TRIGGER_MODE", "Descriptive Name"="MILSTD Trigger Mode", "Data Type"=0, "Command"="TRIG:A:MILS:MODE", "Access"=2, "Range Table"="rsrtx_rngMILSTDTriggerType", "Read Callback"="", "Write Callback"="", "Supported Models"="RTM|RTA", "Instrument Options"="", "Flags"=0, "Help"="Selects the trigger mode.\n\nAvailable Repeated Capabilities:\nNone\n\nRemote-control command(s):\nTRIGger:A:MILStd:MODE"}, {"Level"=3, "Class Only"=FALSE, "Identifier"="RSRTX_ATTR_MILSTD_TRIGGER_SYNCHRONIZATION", "Descriptive Name"="MILSTD Trigger Synchronization", "Data Type"=0, "Command"="TRIG:A:MILS:SYNC", "Access"=2, "Range Table"="rsrtx_rngMILSTDTriggerSync", "Read Callback"="", "Write Callback"="", "Supported Models"="RTM|RTA", "Instrument Options"="", "Flags"=0, "Help"="Selects the trigger type.\n\nAvailable Repeated Capabilities:\nNone\n\nRemote-control command(s):\nTRIGger:A:MILStd:SYNC"}, {"Level"=3, "Class Only"=FALSE, "Identifier"="RSRTX_ATTR_MILSTD_TRIGGER_WORD", "Descriptive Name"="MILSTD Trigger Word", "Data Type"=0, "Command"="TRIG:A:MILS:WORD", "Access"=2, "Range Table"="rsrtx_rngMILSTDTriggerWord", "Read Callback"="", "Write Callback"="", "Supported Models"="RTM|RTA", "Instrument Options"="", "Flags"=0, "Help"="Selects the word type to be triggered on.\n\nAvailable Repeated Capabilities:\nNone\n\nRemote-control command(s):\nTRIGger:A:MILStd:WORD"}, {"Level"=3, "Class Only"=FALSE, "Identifier"="RSRTX_ATTR_MILSTD_TRIGGER_TRANSMISSION_TYPE", "Descriptive Name"="MILSTD Trigger Transmission Type", "Data Type"=0, "Command"="TRIG:A:MILS:TTYP", "Access"=2, "Range Table"="rsrtx_rngMILSTDTransmissionType", "Read Callback"="", "Write Callback"="", "Supported Models"="RTM|RTA", "Instrument Options"="", 
